vi "READ - Wave File.vi"(0 "reference in":refnum<class "WaveFile.lvclass">, 5 "error in (no error)":errorcluster, 7 "Wave File Path - READ":path, 9 "Channel Offset (0 => ignore)":i32) -> (14 "reference out":refnum<class "WaveFile.lvclass">, 19 "error out":errorcluster)   [LabVIEW 2020, in "WaveFile.lvclass"]
uses:
  WaveFile.lvclass
  API/GSwFormDSP_class/functions/Attribute List.ctl
  API/GSwFormDSP_class/GSwFormDSP.lvclass
  API/Generic Utilities_class/Generic Utilities.lvclass
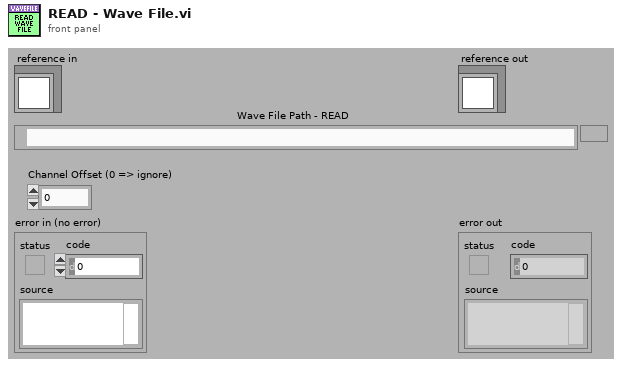
[diagram p1: front panel]
types:
  T1 = typedef "GSwFormDSP.lvclass/Attribute List.ctl" = string
  T2 = typedef "WaveFile.lvclass/ObjectAttributesRef.ctl" = refnum<data-value>
  T3 = typedef "WaveFile.lvclass/ObjectAttributes.ctl" = cluster{"Time Data":refnum<class "GSwFormDSP.lvclass">, "New Time Data Obj?":bool, "NIST File Header":T4}
  T4 = typedef "WaveFile.lvclass/NIST File Header.ctl" = cluster{"Version":string, "Header Nb Bytes":i32, "Nb Samples":i32, "Nb Bytes/sample":i32, "Nb Channels":i32, "byte order":enum16{"big-endian, network order", "native, host order", "little-endian"}, "Fs":dbl, "Valid Header?":bool}
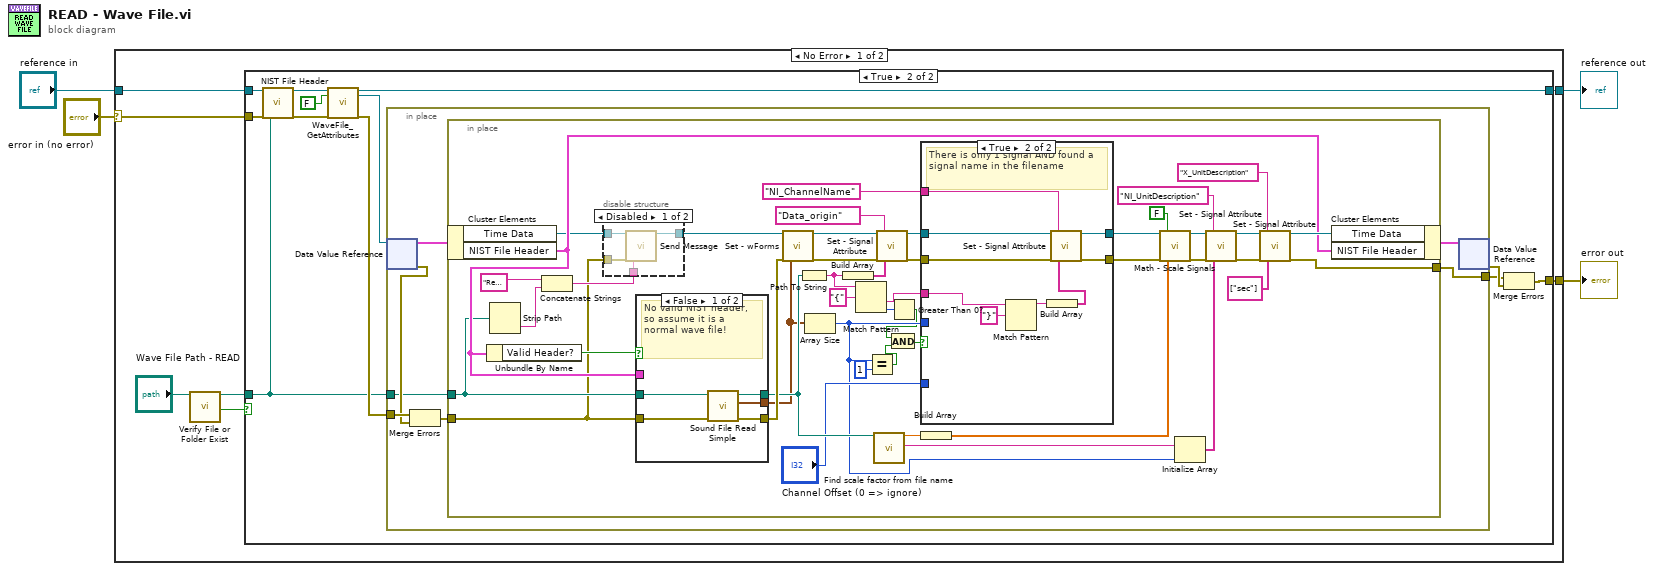
[diagram p0: block diagram]
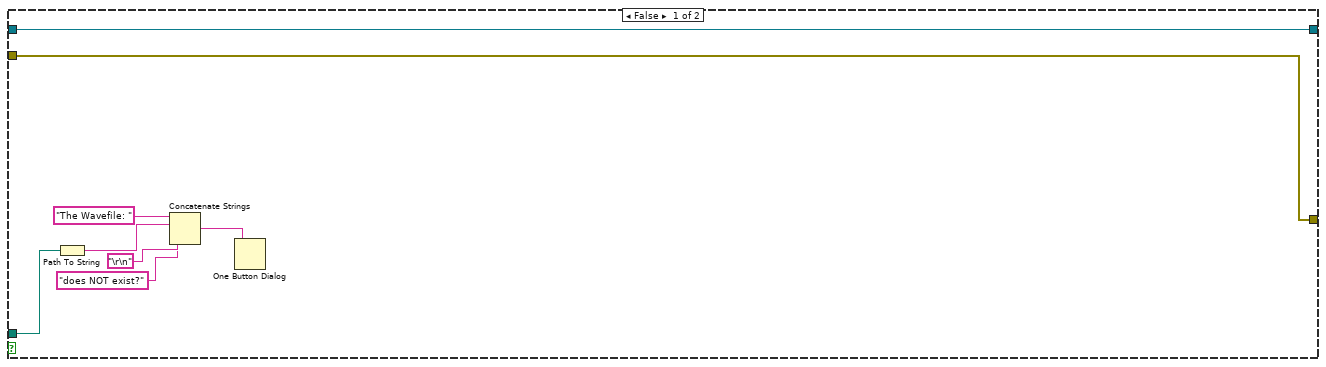
[diagram p2: hidden frame]
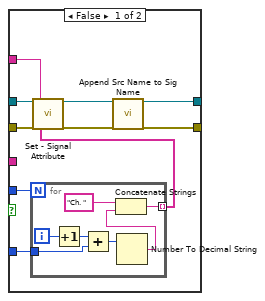
[diagram p4: hidden frame]
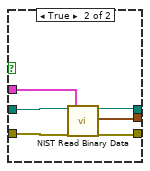
[diagram p5: hidden frame]
diagram:
  n1 = case shown="No Error" "error in (no error)" {
    selector: "error in (no error)" -> [w9 w127]
    tunnel: [w11 w127] -> w3
    tunnel: [w8 w126] -> w1
    tunnel: "reference in" -> [w10 w126]
    frame No Error {
      n2 = call "Verify File or Folder Exist.vi"("path"="Wave File Path - READ") -> ("dup path"=w5:path, "file or folder exists?"=w6:bool)  [unwired: 16 in, 1 out]
      n3 = case shown="True" w6 {
        tunnel: [w13 w31] -> w11
        tunnel: w10 -> [w14 w25]
        tunnel: w9 -> [w13 w23]
        tunnel: [w14 w27] -> w8
        tunnel: w5 -> [w15 w20]
        frame False {
          n4 = Path To String(path=w15) -> (string=w19:string)
          n5 = Concatenate Strings("The Wavefile: ", w19, "\r\n", "does NOT exist?") -> (w16:string)
          n6 = One Button Dialog(message=w16) -> ()  [unwired: 1 in, 1 out]
        }
        frame True {
          n7 = call "NIST File Header.vi"("reference in"=w25, "error in (no error)"=w23, "Wave File Path - READ"=w20) -> ("reference out"=w24:refnum<class "WaveFile.lvclass">, "error out"=w22:errorcluster)  [unwired: 15 in]
          n8 = call "WaveFile_GetAttributes.vi"("reference in"=w24, "return data? (T)"=FALSE, "error in (no error)"=w22) -> ("reference out"=w27:refnum<class "WaveFile.lvclass">, "attributes ref"=w26:T2, "error out"=w21:errorcluster)  [unwired: 13 in, 1 out]
          n9 = in-place {
            in-place-border: [w36] -> w29
            in-place-border: w21 -> [w35]
            in-place-border: w20 -> [w32]
            n10 = in-place-dvr #1(w26) -> (w37:T3, w33:errorcluster)
            n11 = Merge Errors(w35, w33) -> (w34:errorcluster)
            n12 = in-place {
              in-place-border: w34 -> [w39]
              in-place-border: [w82] -> w36
              in-place-border: w32 -> [w50]
              n13 = in-place-cluster #2(w37) -> ("Time Data"=w52:refnum<class "GSwFormDSP.lvclass">, "NIST File Header"=w59:T4)
              n14 = Unbundle By Name(w59) -> ("Valid Header?"=w60:bool)
              n15 = Strip Path(path=w50) -> (name=w54:string)  [unwired: 1 out]
              n16 = Concatenate Strings("Reading File => ", w54) -> (w53:string)
              n17 = disable-structure shown="Disabled" {
                disable-tunnel: w53 -> [w87 _]
                disable-tunnel: w52 -> [w86 w88]
                disable-tunnel: [w85 w88] -> w51
                disable-tunnel: w39 -> [w84 _]
                frame Disabled {
                  n18 = call-dynamic "Send Message.vi"("reference in"=w86, "error in (no error)"=w84, "Message (\"\" closes the window)"=w87) -> ("reference out"=w85:refnum<class "GSwFormDSP.lvclass">)  [unwired: 15 in, 1 out]
                }
                frame Enabled {
                }
              }
              n19 = case shown="False" w60 {
                tunnel: w39 -> [w119 w124]
                tunnel: [w118 w122] -> w81
                tunnel: [w117 w120] -> w56
                tunnel: [w116 w123] -> w71
                tunnel: w50 -> [w115 w125]
                tunnel: w59 -> [_ w121]
                frame False {
                  # "No valid NIST header, so assume it is a normal wave file!"
                  n20 = call <vilib>:"Sound File Read Simple.vi"("error in (no error)"=w119, "path"=w115) -> ("error out"=w118:errorcluster, "data"=w117:waveform(dbl)[], "path out"=w116:path)  [unwired: 6 in, 1 out]
                }
                frame True {
                  n21 = call "NIST Read Binary Data.vi"("Wave File Path IN"=w125, "error in (no error)"=w124, "NIST File Header"=w121) -> ("Wave File Path OUT"=w123:path, "Data"=w120:waveform(dbl)[], "error out"=w122:errorcluster)  [unwired: 14 in]
                }
              }
              n22 = call "Set - wForms.vi"("reference in"=w51, "error in (no error)"=w81, "wForms"=w56) -> ("reference out"=w80:refnum<class "GSwFormDSP.lvclass">, "error out"=w79:errorcluster)  [unwired: 15 in]
              n23 = Path To String(path=w71) -> (string=w48:string)
              n24 = Array Size(array=w56) -> (size(s)=w45:i32)
              n25 = Build Array(w48) -> (w70:string[])
              n26 = Match Pattern(string=w48, regular expression="{") -> (after substring=w40:string, offset past match=w46:i32)  [unwired: 1 in, 2 out]
              n27 = Equal?(x=w45, y=1) -> (x = y?=w41:bool)
              n28 = call "Find scale factor from file name.vi"("Wave File Path - READ"=w71) -> ("Scale Factor"=w77:dbl, "Unit"=w73:string)  [unwired: 17 in]
              n29 = call-dynamic "Set - Signal Attribute.vi"("reference in"=w80, "error in (no error)"=w79, "wForm Attributes"=T1 "Data_origin", "Attribute"=w70) -> ("reference in"=w68:refnum<class "GSwFormDSP.lvclass">, "error out"=w67:errorcluster)  [unwired: 14 in]
              n30 = Greater Than 0?(x=w46) -> (x > 0?=w42:bool)
              n31 = And(x=w42, y=w41) -> (x .and. y?=w43:bool)
              n32 = case shown="True" w43 {
                tunnel: w68 -> [w98 w113]
                tunnel: w67 -> [w97 w112]
                tunnel: T1 "NI_ChannelName" ("wForm Attributes") -> [w96 w114]
                tunnel: [w93 w110] -> w58
                tunnel: [w92 w111] -> w57
                tunnel: w45 -> [w91 _]
                tunnel: "Channel Offset (0 => ignore)" -> [w89 _]
                tunnel: w40 -> [_ w106]
                frame False {
                  n33 = for {
                    N: w91 -> [_]
                    tunnel: [w102] -> w90 mode=indexing
                    tunnel: w89 -> [w99]
                    i -> [w105]
                    n34 = Increment(x=w105) -> (x+1=w101:i32)
                    n35 = Add(x=w101, y=w99) -> (x+y=w100:i32)
                    n36 = Number To Decimal String(number=w100) -> (decimal integer string=w103:string)  [unwired: 1 in]
                    n37 = Concatenate Strings("Ch. ", w103) -> (w102:string)
                  }
                  n38 = call-dynamic "Set - Signal Attribute.vi"("reference in"=w98, "error in (no error)"=w97, "wForm Attributes"=w96, "Attribute"=w90) -> ("reference in"=w95:refnum<class "GSwFormDSP.lvclass">, "error out"=w94:errorcluster)  [unwired: 14 in]
                  n39 = call "Append Src Name to Sig Name.vi"("reference in"=w95, "error in (no error)"=w94) -> ("reference out"=w93:refnum<class "GSwFormDSP.lvclass">, "error out"=w92:errorcluster)  [unwired: 16 in]
                }
                frame True {
                  # "There is only 1 signal AND found a signal name in the filename"
                  n40 = Match Pattern(string=w106, regular expression="}") -> (before substring=w108:string)  [unwired: 1 in, 3 out]
                  n41 = Build Array(w108) -> (w107:string[])
                  n42 = call-dynamic "Set - Signal Attribute.vi"("reference in"=w113, "error in (no error)"=w112, "wForm Attributes"=w114, "Attribute"=w107) -> ("reference in"=w110:refnum<class "GSwFormDSP.lvclass">, "error out"=w111:errorcluster)  [unwired: 14 in]
                }
              }
              n43 = Build Array(w77) -> (w76:dbl[])
              n44 = call-dynamic "Math - Scale Signals.vi"("reference in"=w58, "error in (no error)"=w57, "Anotate Signal Name"=FALSE, "Scaling Factors"=w76) -> ("reference in"=w75:refnum<class "GSwFormDSP.lvclass">, "error out"=w74:errorcluster)  [unwired: 14 in]
              n45 = Initialize Array(w73, w45) -> (w72:string[])
              n46 = call-dynamic "Set - Signal Attribute.vi"("reference in"=w75, "error in (no error)"=w74, "wForm Attributes"=T1 "NI_UnitDescription", "Attribute"=w72) -> ("reference in"=w63:refnum<class "GSwFormDSP.lvclass">, "error out"=w64:errorcluster)  [unwired: 14 in]
              n47 = call-dynamic "Set - Signal Attribute.vi"("reference in"=w63, "error in (no error)"=w64, "wForm Attributes"=T1 "X_UnitDescription", "Attribute"=string[] ["sec"]) -> ("reference in"=w83:refnum<class "GSwFormDSP.lvclass">, "error out"=w82:errorcluster)  [unwired: 14 in]
              n48 = in-place-cluster #2("Time Data"=w83, "NIST File Header"=w59) -> (w38:T3)
            }
            n49 = in-place-dvr #1(w38) -> (w30:errorcluster)  [unwired: 1 out]
          }
          n50 = Merge Errors(w29, w30) -> (w31:errorcluster)
        }
      }
    }
    frame Error {
    }
  }
  "error out" <- w3
  "reference out" <- w1
